vi "QueueOutJAPC.vi"() -> ()   [LabVIEW 2014]
panel:
  in  "Stop Button":bool
  out "data":dbl
  out "error out":errorcluster
  in  "error in (no error)":errorcluster
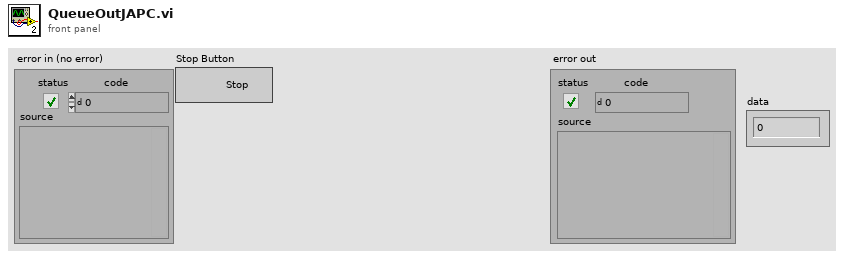
[diagram p1: front panel]
types:
  T1 = typedef "DataQueue1Cluster.ctl" = cluster{"variant":variant, "Enum":T2}
  T2 = typedef "DataQueue1Enum.ctl" = enum16{"Display", "Store"}
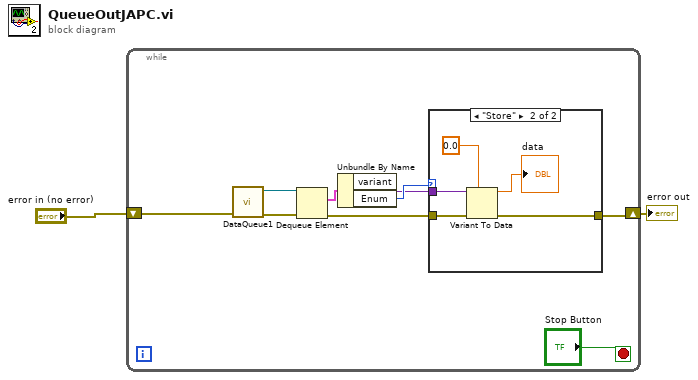
[diagram p0: block diagram]
diagram:
  n1 = while {
    shift-right: [w5] -> w2
    shift-left: "error in (no error)" -> [w4]
    stop <- "Stop Button" stop-if-true
    n2 = call "DataQueue1.vi"("error in"=w4) -> ("error out"=w6:errorcluster, "queue out"=w7:refnum<queue>)  [unwired: 8 in]
    n3 = Dequeue Element(queue=w7, error in (no error)=w6) -> (element=w8:T1, error out=w10:errorcluster)  [unwired: 1 in, 2 out]
    n4 = Unbundle By Name(w8) -> ("variant"=w9:variant, "Enum"=w11:T2)
    n5 = case shown="\"Store\"" w11 {
      tunnel: w9 -> [_ w17]
      tunnel: w10 -> [w12 w15]
      tunnel: [w12 w14] -> w5
      frame "Display", Default {
      }
      frame "Store" {
        n6 = Variant To Data(error in=w15, type=0.0, Variant=w17) -> (data=→"data":dbl, error out=w14:errorcluster)
      }
    }
  }
  "error out" <- w2
